vi "TriggerRotateLogic.vi"(9 "Deadband":dbl, 10 "Right Trigger":dbl, 11 "Left Trigger":dbl) -> (3 "Output":dbl)   [LabVIEW 2014]
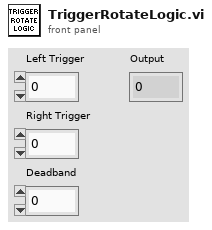
[diagram p1: front panel]
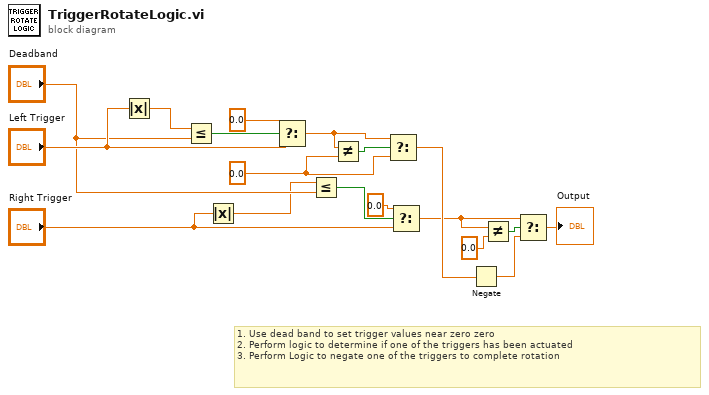
[diagram p0: block diagram]
diagram:
  w13 = 0.0 ("y")
  # "1. Use dead band to set trigger values near zero zero\n2. Perform logic to determine if one of the triggers has been actuated\n3. Perform Logic to negate one of the triggers to complete rotation"
  n1 = Absolute Value(x="Left Trigger") -> (abs(x)=w1:dbl)
  n2 = Less Or Equal?(x=w1, y="Deadband") -> (x <= y?=w4:bool)
  n3 = Absolute Value(x="Right Trigger") -> (abs(x)=w2:dbl)
  n4 = Select(t=0.0, s=w4, f="Left Trigger") -> (s? t:f=w14:dbl)
  n5 = Less Or Equal?(x=w2, y="Deadband") -> (x <= y?=w7:bool)
  n6 = Not Equal?(x=w14, y=w13) -> (x != y?=w12:bool)
  n7 = Select(t=w14, s=w12, f=w13) -> (s? t:f=w17:dbl)
  n8 = Select(t=0.0, s=w7, f="Right Trigger") -> (s? t:f=w15:dbl)
  n9 = Negate(x=w17) -> (-x=w18:dbl)
  n10 = Not Equal?(x=w15, y=0.0) -> (x != y?=w11:bool)
  n11 = Select(t=w15, s=w11, f=w18) -> (s? t:f=→"Output":dbl)
